vi "RT_Gravitational_Force_in_DLR_Navigation_Reference_System_2 (SubVI).vi"(0 "Data":dbl[][](array[numeric]), 5 "i":i32, 9 "input cluster":T1) -> (4 "FG_d":dbl[](array[numeric]), 15 "L_C (rad)":dbl)   [LabVIEW 2017]
panel:
  out "M":dbl
  out "gl_tC":dbl
  out "gl_rC":dbl
  out "R_l (m)":dbl
  out "D_l":dbl
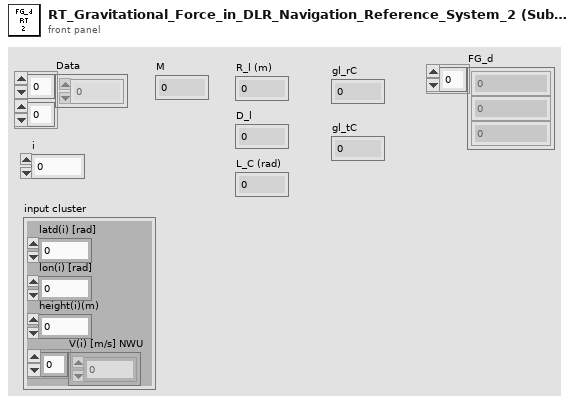
[diagram p1: front panel]
types:
  T1 = cluster{"latd(i) [rad]":dbl, "lon(i) [rad]":dbl, "height(i)(m)":dbl, "V(i) [m/s] NWU":dbl[]}
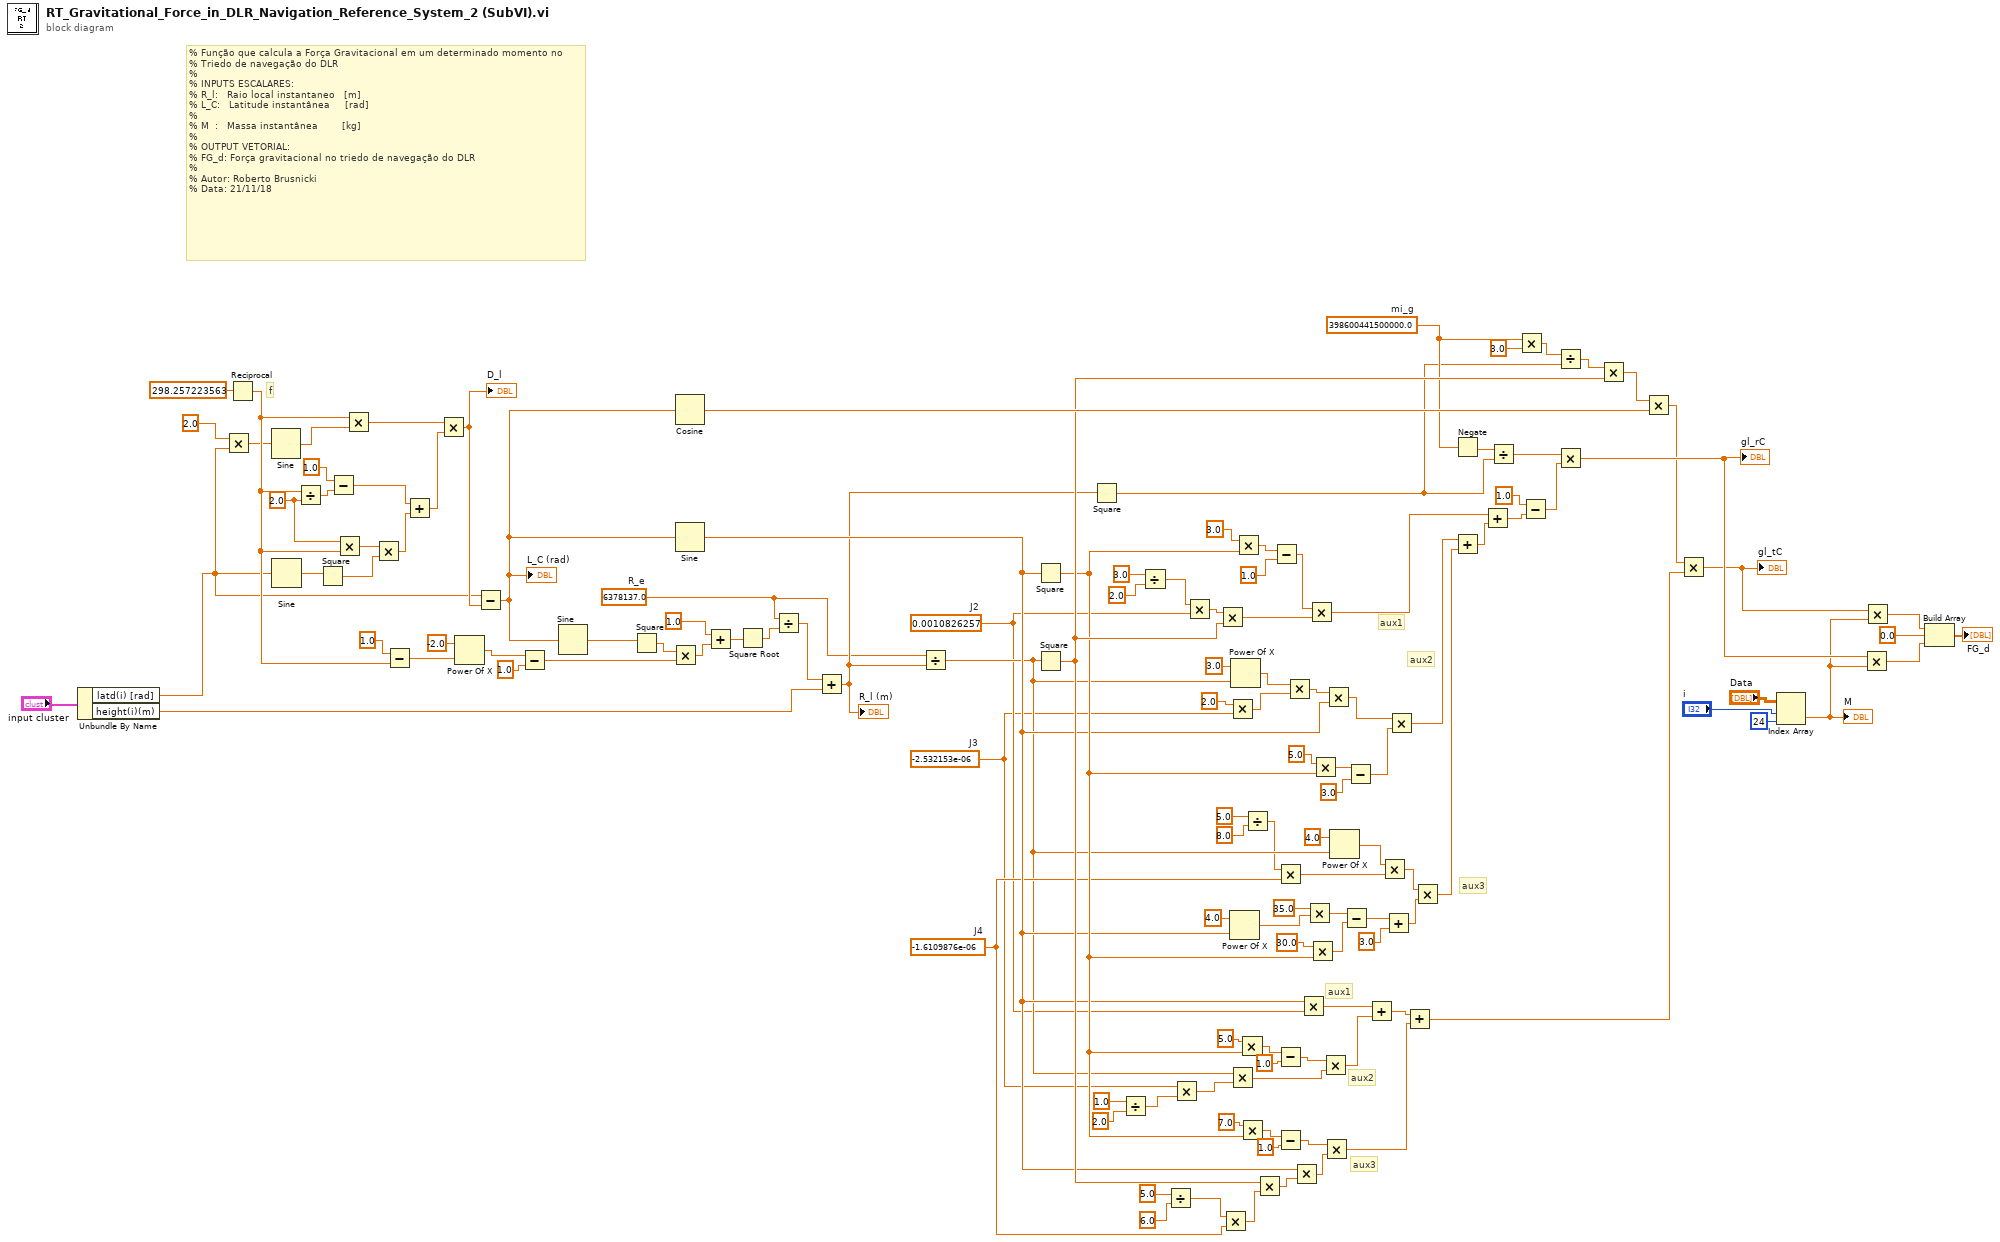
[diagram p0: block diagram]
diagram:
  w94 = -1.6109876e-06  # J4
  w11 = -2.532153e-06  # J3
  w83 = 0.0010826257  # J2
  w105 = 398600441500000.0  # mi_g
  w15 = 2.0 ("y")
  w46 = 6378137.0  # R_e
  # "f"
  # "aux3"
  # "aux2"
  # "aux1"
  # "aux3"
  # "aux2"
  # "aux1"
  # "% Função que calcula a Força Gravitacional em um determinado momento no \n% Triedo de navegação do DLR\n%\n% INPUTS ESCALARES: \n% R_l:   Raio local instantaneo   [m]\n% L_C:   Latitude instantânea     [rad]\n% \n% M  :   Massa instantânea        [kg]\n%\n% OUTPUT VETORIAL:\n% FG_d: Força gravitacional no triedo de navegação do DLR\n%\n% Autor: Roberto Brusnicki\n% Data: 21/11/18"
  n1 = Unbundle By Name("input cluster") -> ("latd(i) [rad]"=w3:dbl, "height(i)(m)"=w2:dbl)
  n2 = Multiply(x=2.0, y=w3) -> (x*y=w18:dbl)
  n3 = Reciprocal(x=298.257223563) -> (1/x=w31:dbl)
  n4 = Sine(x=w18) -> (sin(x)=w19:dbl)
  n5 = Sine(x=w3) -> (sin(x)=w23:dbl)
  n6 = Divide(x=w31, y=w15) -> (x/y=w21:dbl)
  n7 = Square(x=w23) -> (x^2=w25:dbl)
  n8 = Subtract(x=1.0, y=w21) -> (x-y=w26:dbl)
  n9 = Multiply(x=w15, y=w31) -> (x*y=w24:dbl)
  n10 = Multiply(x=w31, y=w19) -> (x*y=w20:dbl)
  n11 = Multiply(x=w24, y=w25) -> (x*y=w27:dbl)
  n12 = Subtract(x=1.0, y=w31) -> (x-y=w32:dbl)
  n13 = Add(x=w26, y=w27) -> (x+y=w28:dbl)
  n14 = Multiply(x=w20, y=w28) -> (x*y=w29:dbl)
  "D_l" <- w29
  n15 = Power Of X(1:w32, 2:-2.0 ("y")) -> (0:w34:dbl)
  n16 = Subtract(x=w3, y=w29) -> (x-y=w112:dbl)
  "L_C (rad)" <- w112
  n17 = Subtract(x=w34, y=1.0) -> (x-y=w39:dbl)
  n18 = Sine(x=w112) -> (sin(x)=w37:dbl)
  n19 = Square(x=w37) -> (x^2=w38:dbl)
  n20 = Multiply(x=w38, y=w39) -> (x*y=w40:dbl)
  n21 = Cosine(x=w112) -> (cos(x)=w111:dbl)
  n22 = Sine(x=w112) -> (sin(x)=w97:dbl)
  n23 = Add(x=1.0, y=w40) -> (x+y=w41:dbl)
  n24 = Square Root(x=w41) -> (sqrt(x)=w42:dbl)
  n25 = Divide(x=w46, y=w42) -> (x/y=w43:dbl)
  n26 = Add(x=w43, y=w2) -> (x+y=w75:dbl)
  "R_l (m)" <- w75
  n27 = Divide(x=w46, y=w75) -> (x/y=w84:dbl)
  n28 = Square(x=w97) -> (x^2=w102:dbl)
  n29 = Square(x=w84) -> (x^2=w108:dbl)
  n30 = Square(x=w75) -> (x^2=w104:dbl)
  n31 = Divide(x=1.0, y=2.0) -> (x/y=w13:dbl)
  n32 = Divide(x=3.0, y=2.0) -> (x/y=w45:dbl)
  n33 = Divide(x=5.0, y=6.0 ("x")) -> (x/y=w91:dbl)
  n34 = Multiply(x=w11, y=w13) -> (x*y=w12:dbl)
  n35 = Multiply(x=w45, y=w83) -> (x*y=w47:dbl)
  n36 = Multiply(x=w47, y=w108) -> (x*y=w48:dbl)
  n37 = Multiply(x=w91, y=w94) -> (x*y=w95:dbl)
  n38 = Multiply(x=2.0, y=w11) -> (x*y=w56:dbl)
  n39 = Multiply(x=w84, y=w12) -> (x*y=w14:dbl)
  n40 = Power Of X(1:w97, 2:4.0 ("y")) -> (0:w69:dbl)
  n41 = Power Of X(1:w84, 2:3.0 ("y")) -> (0:w55:dbl)
  n42 = Multiply(x=3.0, y=w102) -> (x*y=w50:dbl)
  n43 = Multiply(x=5.0, y=w102) -> (x*y=w88:dbl)
  n44 = Multiply(x=7.0, y=w102) -> (x*y=w100:dbl)
  n45 = Divide(x=5.0, y=8.0 ("x")) -> (x/y=w63:dbl)
  n46 = Multiply(x=w108, y=w95) -> (x*y=w96:dbl)
  n47 = Subtract(x=w50, y=1.0) -> (x-y=w52:dbl)
  n48 = Multiply(x=w63, y=w94) -> (x*y=w66:dbl)
  n49 = Subtract(x=w88, y=1.0) -> (x-y=w90:dbl)
  n50 = Subtract(x=w100, y=1.0) -> (x-y=w98:dbl)
  n51 = Multiply(x=w55, y=w56) -> (x*y=w57:dbl)
  n52 = Multiply(x=w97, y=w96) -> (x*y=w103:dbl)
  n53 = Multiply(x=w97, y=w83) -> (x*y=w113:dbl)
  n54 = Multiply(x=35.0, y=w69) -> (x*y=w70:dbl)
  n55 = Multiply(x=w52, y=w48) -> (x*y=w78:dbl)
  n56 = Multiply(x=30.0, y=w102) -> (x*y=w6:dbl)
  n57 = Multiply(x=5.0, y=w102) -> (x*y=w9:dbl)
  n58 = Multiply(x=w90, y=w14) -> (x*y=w114:dbl)
  n59 = Multiply(x=w98, y=w103) -> (x*y=w116:dbl)
  n60 = Multiply(x=w57, y=w97) -> (x*y=w58:dbl)
  n61 = Power Of X(1:w84, 2:4.0 ("y")) -> (0:w65:dbl)
  n62 = Subtract(x=w70, y=w6) -> (x-y=w5:dbl)
  n63 = Subtract(x=w9, y=3.0) -> (x-y=w8:dbl)
  n64 = Add(x=w113, y=w114) -> (x+y=w115:dbl)
  n65 = Multiply(x=w65, y=w66) -> (x*y=w73:dbl)
  n66 = Add(x=w5, y=3.0) -> (x+y=w4:dbl)
  n67 = Multiply(x=w58, y=w8) -> (x*y=w7:dbl)
  n68 = Add(x=w115, y=w116) -> (x+y=w118:dbl)
  n69 = Multiply(x=w73, y=w4) -> (x*y=w79:dbl)
  n70 = Negate(x=w105) -> (-x=w74:dbl)
  n71 = Add(x=w7, y=w79) -> (x+y=w80:dbl)
  n72 = Add(x=w78, y=w80) -> (x+y=w77:dbl)
  n73 = Divide(x=w74, y=w104) -> (x/y=w81:dbl)
  n74 = Multiply(x=w105, y=3.0) -> (x*y=w107:dbl)
  n75 = Subtract(x=1.0, y=w77) -> (x-y=w82:dbl)
  n76 = Divide(x=w107, y=w104) -> (x/y=w109:dbl)
  n77 = Multiply(x=w81, y=w82) -> (x*y=w126:dbl)
  "gl_rC" <- w126
  n78 = Multiply(x=w109, y=w108) -> (x*y=w110:dbl)
  n79 = Multiply(x=w110, y=w111) -> (x*y=w117:dbl)
  n80 = Multiply(x=w117, y=w118) -> (x*y=w124:dbl)
  "gl_tC" <- w124
  n81 = Index Array(array="Data", index (row)="i", index (col)=24 ("disabled index (col)")) -> (element=w123:dbl)
  "M" <- w123
  n82 = Multiply(x=w126, y=w123) -> (x*y=w127:dbl)
  n83 = Multiply(x=w124, y=w123) -> (x*y=w125:dbl)
  n84 = Build Array(w125, 0.0 ("y"), w127) -> (→"FG_d":dbl[])
